vi "get_current_RGB_image.vi"(8 "error in (no error)":errorcluster, 11 "GenericDisplay in":refnum<class "GenericDisplay.lvclass">) -> (0 "error out":errorcluster, 2 "RGB image":refnum<class "Image.lvclass">, 3 "GenericDisplay out":refnum<class "GenericDisplay.lvclass">)   [LabVIEW 2010, in "GenericDisplay.lvclass"]
uses:
  GenericDisplay.lvclass
  common/classes/Image/Image/Image.lvclass
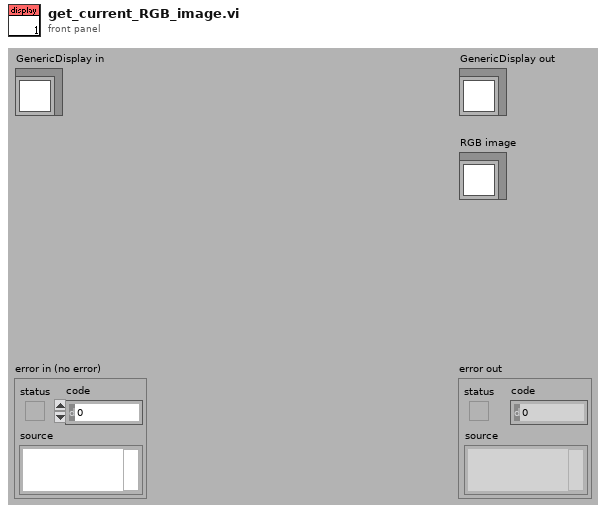
[diagram p1: front panel]
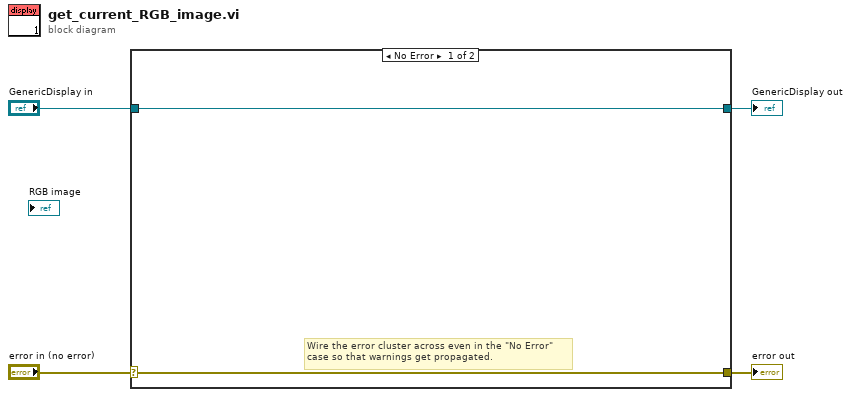
[diagram p0: block diagram]
diagram:
  n1 = case shown="No Error" "error in (no error)" {
    selector: "error in (no error)" -> [w5 w8]
    tunnel: [w5 w8] -> w3
    tunnel: [w6 w7] -> w1
    tunnel: "GenericDisplay in" -> [w6 w7]
    frame No Error {
      # "Wire the error cluster across even in the \"No Error\"\ncase so that warnings get propagated."
    }
    frame Error {
    }
  }
  "error out" <- w3
  "GenericDisplay out" <- w1
